vi "Toggle Emergency.vi"(11 "AT Command Port":refnum<k16>) -> (3 "AT Command Port":refnum<k16>)   [LabVIEW 2011]
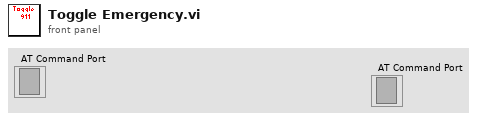
[diagram p1: front panel]
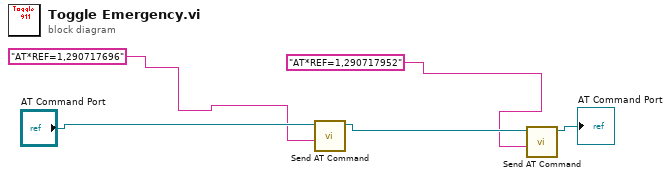
[diagram p0: block diagram]
diagram:
  n1 = call "Send AT Command.vi"("AT Command"="AT*REF=1,290717696", "AT Command Port"="AT Command Port") -> ("AT Command Port"=w4:refnum<k16>)  [unwired: 9 in]
  n2 = call "Send AT Command.vi"("AT Command"="AT*REF=1,290717952", "AT Command Port"=w4) -> ("AT Command Port"=→"AT Command Port":refnum<k16>)  [unwired: 9 in]
